vi "ad set trigger pos.vi"(8 "error in (no error)":errorcluster, 10 "pos":cluster{"run":u32, "offset":u32}, 11 "adh":i32) -> (0 "error out":errorcluster, 2 "pos out":cluster{"run":u32, "offset":u32}, 3 "function return":i32)   [LabVIEW 2021, in "libad4.lvlib"]
doc: "ad_set_trigger_pos (int32_t adh, struct ad_scan_pos *pos);"
uses:
  <userlib>/libad4/libad4.lvlib
  <userlib>/libad4/libad4.dll
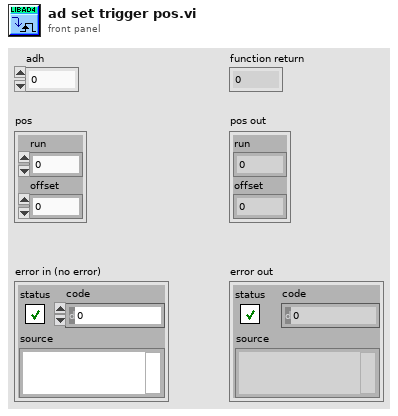
[diagram p1: front panel]
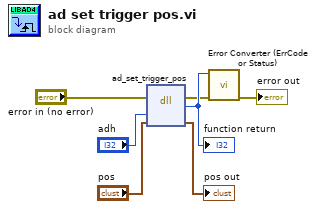
[diagram p0: block diagram]
diagram:
  n1 = dll-call lib="C:/Program Files/National Instruments/LabVIEW 2021/user.lib/libad4/libad4.*" fn="ad_set_trigger_pos"(error in="error in (no error)", "adh"="adh", "pos"="pos") -> (error out=w2:errorcluster, w7:i32, "pos"=→"pos out":cluster{"run":u32, "offset":u32})  [unwired: 3 in, 1 out]
  "function return" <- w7
  n2 = call <userlib>:"Error Converter (ErrCode or Status).vi"("error in (no error)"=w2, "error code"=w7) -> ("error out"=→"error out":errorcluster)  [unwired: 9 in]
